vi "Calculate MCL scan parameters.vi"(0 "Input parameters":T1) -> (1 "Scan steps(MCL)":dbl, 2 "Scan Freq. Increment (MCL)":dbl, 3 "MCL Count":dbl)   [LabVIEW 2014]
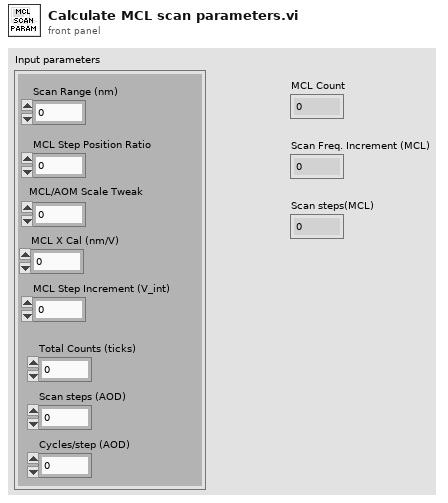
[diagram p1: front panel]
types:
  T1 = cluster{"MCL Step Position Ratio":dbl, "MCL/AOM Scale Tweak":dbl, "MCL X Cal (nm/V)":dbl, "MCL Step Increment (V_int)":dbl, "Scan Range (nm)":dbl, "Total Counts (ticks)":u16, "Scan steps (AOD)":u64, "Cycles/step (AOD)":u64}
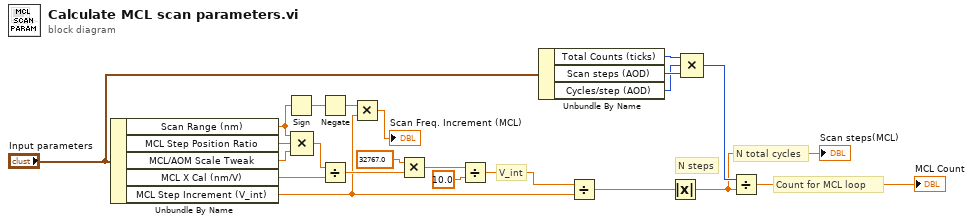
[diagram p0: block diagram]
diagram:
  # "Count for MCL loop"
  # "N total cycles"
  # "N steps"
  # "V_int"
  n1 = Unbundle By Name("Input parameters") -> ("Scan Range (nm)"=w12:dbl, "MCL Step Position Ratio"=w11:dbl, "MCL/AOM Scale Tweak"=w10:dbl, "MCL X Cal (nm/V)"=w8:dbl, "MCL Step Increment (V_int)"=w9:dbl)
  n2 = Sign(1:w12) -> (0:w14:dbl)
  n3 = Compound Arithmetic op=MULTIPLY(w12, w11, w10) -> (w15:dbl)
  n4 = Negate(x=w14) -> (-x=w13:dbl)
  n5 = Divide(x=w15, y=w8) -> (x/y=w19:dbl)
  n6 = Multiply(x=w13, y=w9) -> (x*y=→"Scan Freq. Increment (MCL)":dbl)
  n7 = Multiply(x=32767.0 ("y"), y=w19) -> (x*y=w22:dbl)
  n8 = Divide(x=w22, y=10.0) -> (x/y=w18:dbl)
  n9 = Unbundle By Name("Input parameters") -> ("Total Counts (ticks)"=w6:u16, "Scan steps (AOD)"=w5:u64, "Cycles/step (AOD)"=w4:u64)
  n10 = Divide(x=w18, y=w9) -> (x/y=w16:dbl)
  n11 = Absolute Value(x=w16) -> (abs(x)=w2:dbl)
  "Scan steps(MCL)" <- w2
  n12 = Compound Arithmetic op=MULTIPLY(w6, w4, w5) -> (w17:u64)
  n13 = Divide(x=w17, y=w2) -> (x/y=→"MCL Count":dbl)
